vi "Enqueue Close Connection.vi"(8 "Error In":errorcluster, 11 "Name":string) -> (0 "Error Out":errorcluster)   [LabVIEW 2019, in "TCP2Foxconn.lvlib"]
uses:
  TCP2Foxconn.lvlib
  Queue/Queue.lvlib
  Data Error Notifier/Data and Error Notifier.lvlib
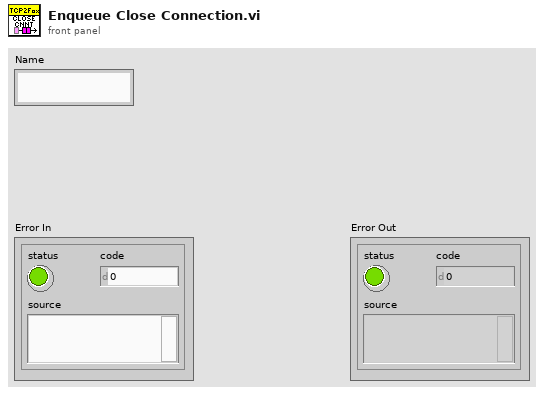
[diagram p1: front panel]
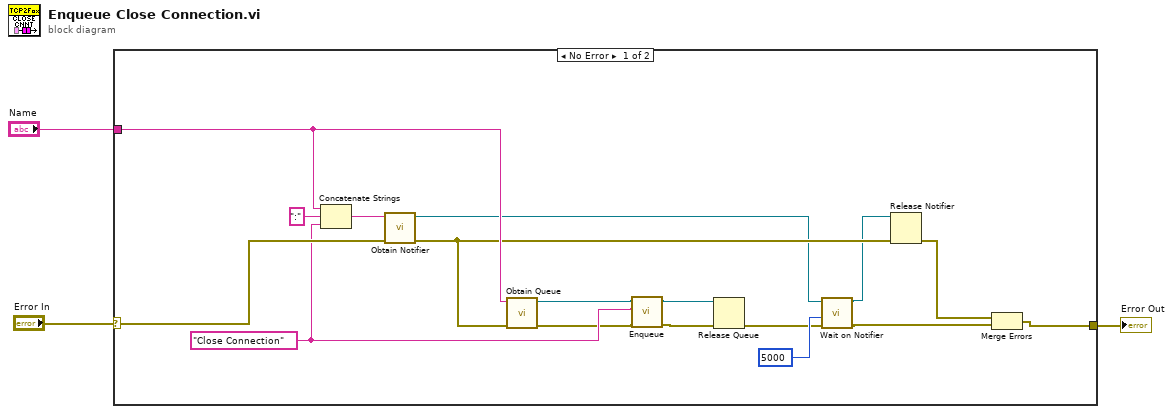
[diagram p0: block diagram]
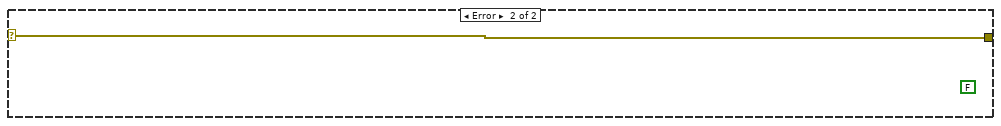
[diagram p2: hidden frame]
diagram:
  n1 = case shown="No Error" "Error In" {
    selector: "Error In" -> [w15 w21]
    tunnel: [w17 w21] -> w2
    tunnel: "Name" -> [w20 _]
    frame No Error {
      w12 = "Close Connection" ("Message")
      n2 = Concatenate Strings(w20, ":" ("string"), w12) -> (w16:string)
      n3 = call "Obtain Notifier.vi"("Error In"=w15, "Name"=w16) -> ("Error Out"=w14:errorcluster, "notifier out"=w8:refnum<notifier>)  [unwired: 8 in]
      n4 = call "Obtain Queue.vi"("Error In"=w14, "Name"=w20) -> ("Error Out"=w11:errorcluster, "queue out"=w13:refnum<queue>)  [unwired: 8 in]
      n5 = call "Enqueue.vi"("Error In"=w11, "Message"=w12, "queue in"=w13) -> ("Error Out"=w9:errorcluster, "queue out"=w10:refnum<queue>)  [unwired: 7 in]
      n6 = Release Queue(queue=w10, error in (no error)=w9) -> (error out=w6:errorcluster)  [unwired: 1 in, 2 out]
      n7 = call "Wait on Notifier.vi"("Error In"=w6, "timeout in ms (-1)"=5000, "notifier in"=w8) -> ("Error Out"=w4:errorcluster, "notifier out"=w5:refnum<notifier>)  [unwired: 6 in, 1 out]
      n8 = Release Notifier(notifier=w5, error in (no error)=w14) -> (error out=w18:errorcluster)  [unwired: 1 in, 2 out]
      n9 = Merge Errors(w18, w4) -> (w17:errorcluster)
    }
    frame Error {
      (unwired) FALSE
    }
  }
  "Error Out" <- w2
